vi "Device Params from Config INI File.vi"(8 "error in":errorcluster, 11 "Configuration in":refnum<class "Configuration.lvclass">) -> (0 "error out":errorcluster, 1 "Device Connections":T5={"PID Connections"={"Integrator DAQ Channels"={"V0"="cDAQ1Mod1/ai0", "S1"="cDAQ1Mod5/port0/line4", "S2"="cDAQ1Mod5/ctr0"}}, "Valve Controller VISA resource name"="COM3", "Detector Connection"=FALSE, "Power Supply Connection"=FALSE, "MFC Connection"=FALSE, "Valve Connection"=FALSE}, 2 "Device Settings":T8, 3 "Configuration out":refnum<class "Configuration.lvclass">)   [LabVIEW 2011]
uses:
  Modules/File/Configuration/Configuration.lvclass
  Controls/Device Settings.ctl
  Modules/Hardware/Power Supply/Source Units.ctl
  Modules/Hardware/Power Supply/Power Supply.lvclass
  Modules/Hardware/Power Supply/Source Mode.ctl
  Modules/Hardware/Mass Flow Controller/Valve Status.ctl
  Modules/Hardware/Mass Flow Controller/Mass Flow Controller.lvclass
  Modules/Hardware/Power Supply/Current Units.ctl
  Modules/Hardware/Power Supply/Voltage Units.ctl
  Modules/Hardware/Power Supply/Protection Limits.ctl
  Modules/Hardware/PID/Integrator DAQmx Channels.ctl
  Modules/Hardware/PID/PID.lvclass
  Modules/Hardware/PID/PID Connections.ctl
  Controls/Device Connections.ctl
  Modules/Hardware/Valve Controller/Valve Assembly.ctl
  Modules/Hardware/Valve Controller/Valve Controller.lvclass
  Controls/Valve Type.ctl
  Modules/File/Configuration/Key Data Type.ctl
  Modules/File/Configuration/PID Keys.ctl
  Modules/File/Configuration/PID Sections.ctl
  Modules/File/Configuration/PID Key Types.ctl
panel:
  in  "Key Types":T1=[enum."I32", enum."I32", enum."I32", enum."I32", enum."I32", enum."I32", enum."I32", enum."I32", enum."I32", enum."I32", enum."Double", enum."Double", enum."Double", enum."Double", enum."Double", enum."Double", enum."Double", enum."Double", enum."Double", enum."Boolean", enum."Boolean", enum."Boolean", enum."DAQmx Channel", enum."DAQmx Channel", enum."DAQmx Channel"]
  in  "Sections":T3=["Devices", "Devices", "Devices", "Devices", "Devices", "Devices", "Devices", "Devices", "Devices", "Devices", "Devices", "Devices", "Devices", "Devices", "Devices", "Devices", "Devices", "Devices", "Devices", "Devices", "Devices", "Devices", "Device Connections", "Device Connections", "Device Connections"]
  in  "Keys":T4=["Detector type", "MFC Type", "PS Type", "PS Source Units", "PS Source Mode", "MFC Valve Status", "PS Voltage Limit Units", "PS Current Limit Units", "PS Voltage Trip/Cmpl Units", "PS Current Trip/Cmpl Units", "PS Source Value", "MFC Flow Rate", "Detector Sampling Frequency", "PS Voltage Limit", "PS Current Limit", "PS Voltage Trip/Cmpl", "PS Current Trip/Cmpl", "PID Grid Voltage", "PID Integration Time", "Detector Connection", "MFC Connection", "PS Connection", "PID Integrator DAQmx Channel V0", "PID Integrator DAQmx Channel S1", "PID Integrator DAQmx Channel S2"]
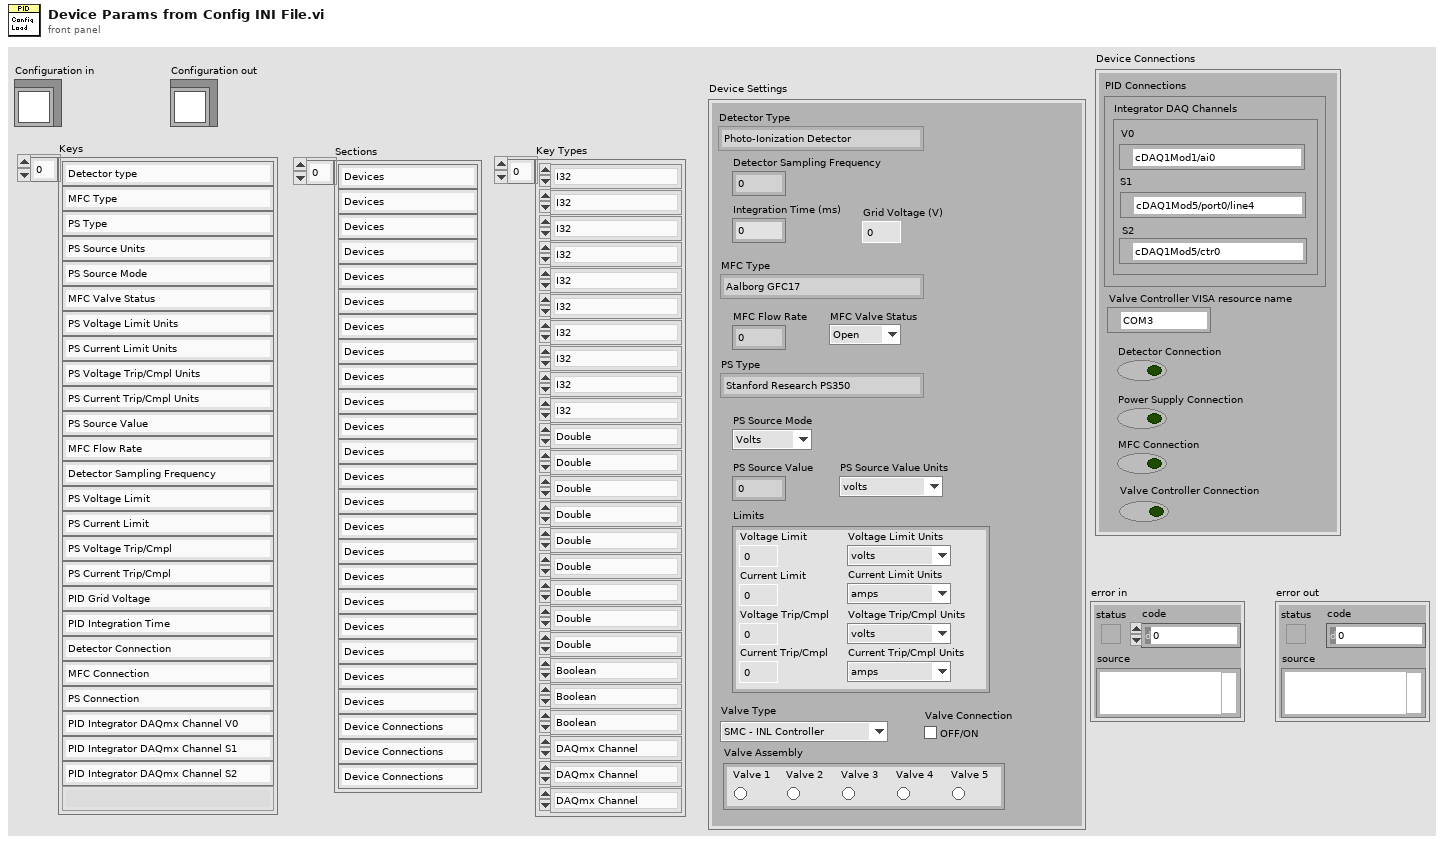
[diagram p1: front panel]
types:
  T1 = typedef "Configuration.lvclass/PID Key Types.ctl" = T2[]
  T2 = typedef "Configuration.lvclass/Key Data Type.ctl" = enum16{"Boolean", "U32", "I32", "Double", "String", "DAQmx Channel", "Path"}
  T3 = typedef "Configuration.lvclass/PID Sections.ctl" = string[]
  T4 = typedef "Configuration.lvclass/PID Keys.ctl" = string[]
  T5 = typedef "Device Connections.ctl" = cluster{"PID Connections":T6, "Valve Controller VISA resource name":refnum<visa-resource-name>, "Detector Connection":bool, "Power Supply Connection":bool, "MFC Connection":bool, "Valve Connection":bool}
  T6 = typedef "PID.lvclass/PID Connections.ctl" = cluster{"Integrator DAQ Channels":T7}
  T7 = typedef "PID.lvclass/Integrator DAQmx Channels.ctl" = cluster{"V0":tag, "S1":tag, "S2":tag}
  T8 = typedef "Device Settings.ctl" = cluster{"Detector Type":enum16{"Photo-Ionization Detector"}, "MFC Type":enum16{"Aalborg GFC17"}, "PS Type":enum16{"Stanford Research PS350", "Keithley 2400"}, "Detector Sampling Frequency":dbl, "MFC Flow Rate":dbl, "MFC Valve Status":T9, "PS Source Mode":T10, "PS Source Value":dbl, "PS Source Value Units":T11, "Limits":T12, "PID Integration Time":dbl, "PID Grid Voltage":dbl, "Valve Type":T15, "Valve Assembly":T16, "Valve Connection":bool}
  T9 = typedef "Mass Flow Controller.lvclass/Valve Status.ctl" = enum16{"Open", "Closed"}
  T10 = typedef "Power Supply.lvclass/Source Mode.ctl" = enum16{"Volts", "Current"}
  T11 = typedef "Power Supply.lvclass/Source Units.ctl" = enum16{"volts", "millivolts", "microvolts", "amps", "milliamps", "microamps", "nanoamps"}
  T12 = typedef "Power Supply.lvclass/Protection Limits.ctl" = cluster{"Voltage Limit":dbl, "Voltage Limit Units":T13, "Current Limit":dbl, "Current Limit Units":T14, "Voltage Trip/Cmpl":dbl, "Voltage Trip/Cmpl Units":T13, "Current Trip/Cmpl":dbl, "Current Trip/Cmpl Units":T14}
  T13 = typedef "Power Supply.lvclass/Voltage Units.ctl" = enum16{"volts", "millivolts", "microvolts"}
  T14 = typedef "Power Supply.lvclass/Current Units.ctl" = enum16{"amps", "milliamps", "microamps", "nanoamps"}
  T15 = typedef "Valve Type.ctl" = enum16{"SMC - INL Controller"}
  T16 = typedef "Valve Controller.lvclass/Valve Assembly.ctl" = cluster{"Valve 1":bool, "Valve 2":bool, "Valve 3":bool, "Valve 4":bool, "Valve 5":bool}
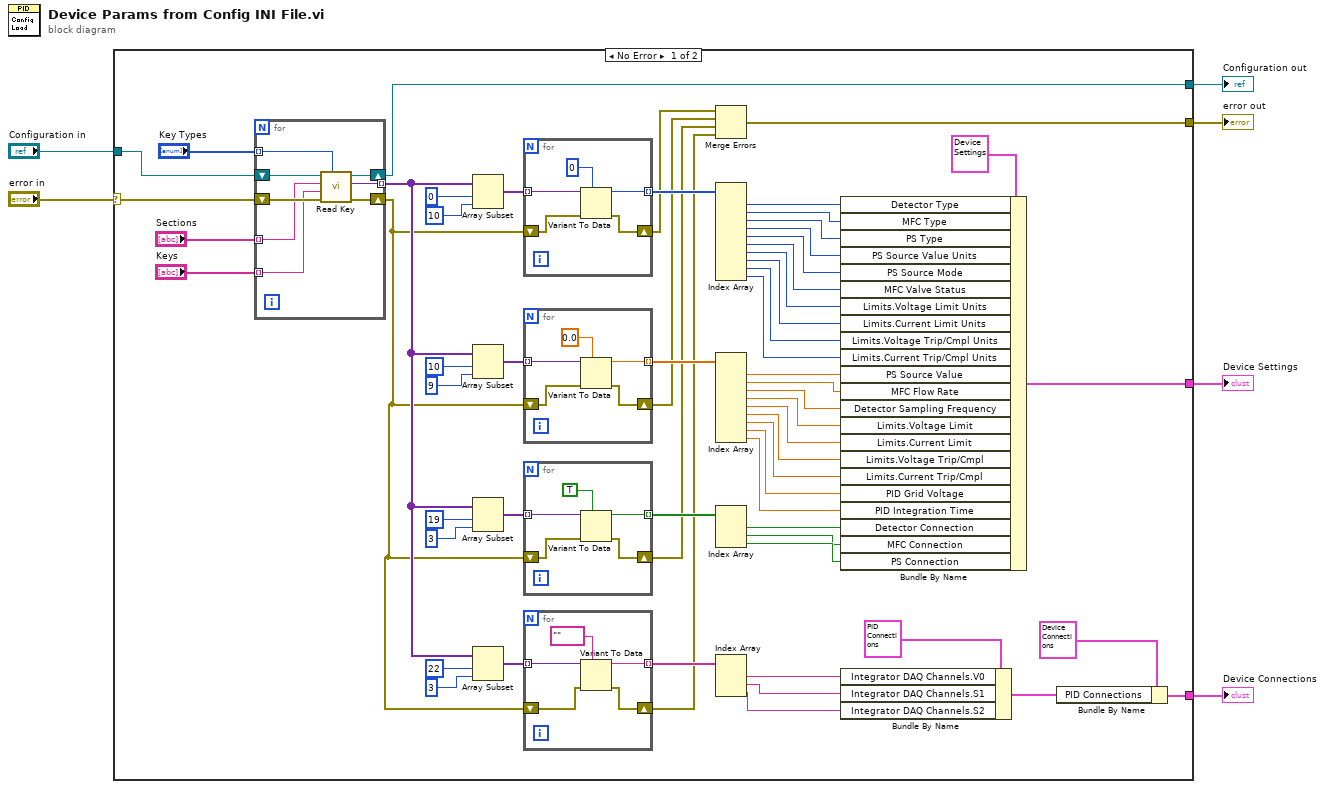
[diagram p0: block diagram]
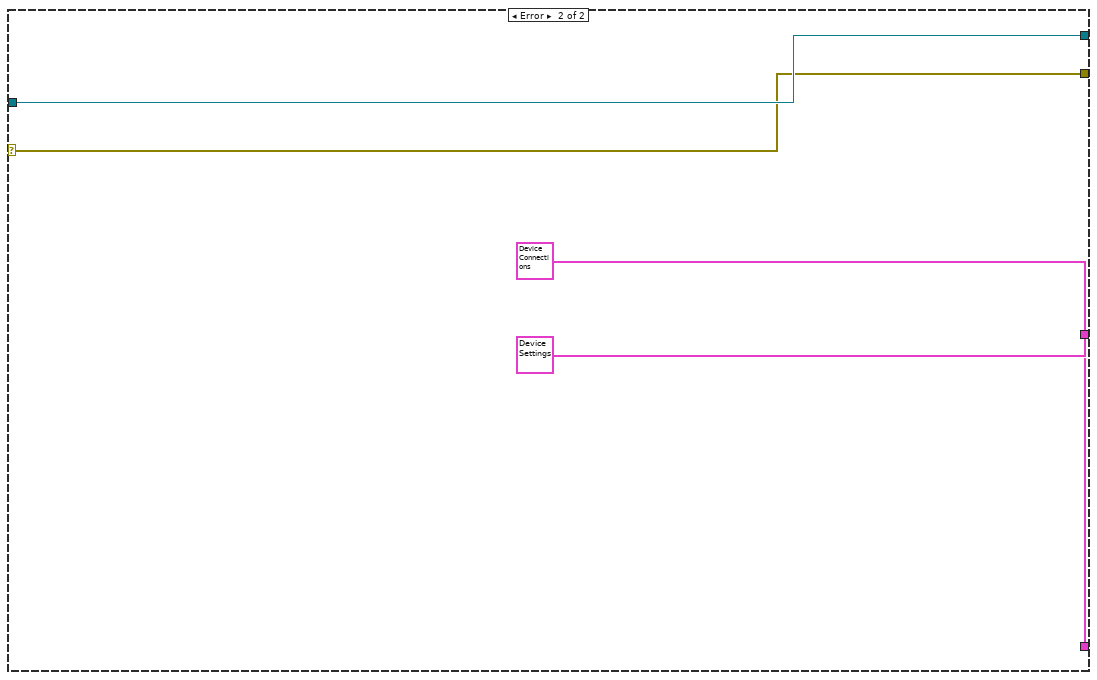
[diagram p2: hidden frame]
diagram:
  n1 = case shown="No Error" "error in" {
    selector: "error in" -> [w66 w97]
    tunnel: [w9 w98] -> w6
    tunnel: "Configuration in" -> [w65 w98]
    tunnel: [w10 w97] -> w4
    tunnel: [w8 T8 {"Detector Type"=enum."Photo-Ionization Detector", "MFC Type"=enum."Aalborg GFC17", "PS Type"=enum."Stanford Research PS350", "Detector Sampling Frequency"=0.0, "MFC Flow Rate"=0.0, "MFC Valve Status"=enum."Open", "PS Source Mode"=enum."Volts", "PS Source Value"=0.0, "PS Source Value Units"=enum."volts", "Limits"={"Voltage Limit"=0.0, "Voltage Limit Units"=enum."volts", "Current Limit"=0.0, "Current Limit Units"=enum."amps", "Voltage Trip/Cmpl"=0.0, "Voltage Trip/Cmpl Units"=enum."volts", "Current Trip/Cmpl"=0.0, "Current Trip/Cmpl Units"=enum."amps"}, "PID Integration Time"=0.0, "PID Grid Voltage"=0.0, "Valve Type"=enum."SMC - INL Controller", "Valve Assembly"={"Valve 1"=FALSE, "Valve 2"=FALSE, "Valve 3"=FALSE, "Valve 4"=FALSE, "Valve 5"=FALSE}, "Valve Connection"=FALSE} ("Device Settings")] -> w2
    tunnel: [w7 T5 {"PID Connections"={"Integrator DAQ Channels"={"V0"="cDAQ1Mod1/ai0", "S1"="cDAQ1Mod5/port0/line4", "S2"="cDAQ1Mod5/ctr0"}}, "Valve Controller VISA resource name"="", "Detector Connection"=FALSE, "Power Supply Connection"=FALSE, "MFC Connection"=FALSE, "Valve Connection"=FALSE} ("Device Connections")] -> w1
    frame No Error {
      n2 = for {
        shift-right: [w93] -> w9
        shift-left: w65 -> [w94]
        shift-right: [w87] -> w15
        shift-left: w66 -> [w92]
        tunnel: [w91] -> w23 mode=indexing
        tunnel: "Sections" -> [w90] mode=indexing
        tunnel: "Keys" -> [w89] mode=indexing
        tunnel: "Key Types" -> [w88] mode=indexing
        n3 = call-dynamic "Read Key.vi"("data type"=w88, "error in (no error)"=w92, "key"=w89, "section"=w90, "Configuration.lvclass in"=w94) -> ("error out"=w87:errorcluster, "Key"=w91:variant, "Configuration.lvclass out"=w93:refnum<class "Configuration.lvclass">)  [unwired: 3 in, 1 out]
      }
      n4 = Array Subset(array=w23, index=0, length=10) -> (w58:variant[])
      n5 = Array Subset(array=w23, index=10, length=9) -> (w44:variant[])
      n6 = Array Subset(array=w23, index=19, length=3) -> (w31:variant[])
      n7 = Array Subset(array=w23, index=22, length=3) -> (w24:variant[])
      n8 = for {
        tunnel: w58 -> [w86] mode=indexing
        tunnel: [w84] -> w57 mode=indexing
        shift-right: [w82] -> w14
        shift-left: w15 -> [w83]
        n9 = Variant To Data(error in=w83, type=0, Variant=w86) -> (data=w84:i32, error out=w82:errorcluster)
      }
      n10 = for {
        tunnel: w44 -> [w81] mode=indexing
        tunnel: [w79] -> w43 mode=indexing
        shift-right: [w77] -> w13
        shift-left: w15 -> [w78]
        n11 = Variant To Data(error in=w78, type=0.0, Variant=w81) -> (data=w79:dbl, error out=w77:errorcluster)
      }
      n12 = for {
        tunnel: w31 -> [w76] mode=indexing
        tunnel: [w75] -> w30 mode=indexing
        shift-right: [w72] -> w12
        shift-left: w15 -> [w73]
        n13 = Variant To Data(error in=w73, type=TRUE, Variant=w76) -> (data=w75:bool, error out=w72:errorcluster)
      }
      n14 = for {
        tunnel: w24 -> [w71] mode=indexing
        tunnel: [w70] -> w20 mode=indexing
        shift-right: [w67] -> w11
        shift-left: w15 -> [w68]
        n15 = Variant To Data(error in=w68, type=tag "" ("Integrator DAQ Channels.V0"), Variant=w71) -> (data=w70:tag, error out=w67:errorcluster)
      }
      n16 = Merge Errors(w14, w13, w12, w11) -> (w10:errorcluster)
      n17 = Index Array(array=w57) -> (element #1=w56:i32, element #2=w55:i32, element #3=w54:i32, element #4=w53:i32, element #5=w47:i32, element #6=w48:i32, element #7=w49:i32, element #8=w50:i32, element #9=w51:i32, element #10=w52:i32)  [unwired: 10 in]
      n18 = Index Array(array=w43) -> (element #1=w42:dbl, element #2=w41:dbl, element #3=w34:dbl, element #4=w35:dbl, element #5=w36:dbl, element #6=w37:dbl, element #7=w38:dbl, element #8=w39:dbl, element #9=w40:dbl)  [unwired: 9 in]
      n19 = Index Array(array=w30) -> (element #1=w29:bool, element #2=w27:bool, element #3=w28:bool)  [unwired: 3 in]
      n20 = Index Array(array=w20) -> (element #1=w19:tag, element #2=w17:tag, element #3=w18:tag)  [unwired: 3 in]
      n21 = Bundle By Name(cluster=T8 {"Detector Type"=enum."Photo-Ionization Detector", "MFC Type"=enum."Aalborg GFC17", "PS Type"=enum."Stanford Research PS350", "Detector Sampling Frequency"=0.0, "MFC Flow Rate"=0.0, "MFC Valve Status"=enum."Open", "PS Source Mode"=enum."Volts", "PS Source Value"=0.0, "PS Source Value Units"=enum."volts", "Limits"={"Voltage Limit"=0.0, "Voltage Limit Units"=enum."volts", "Current Limit"=0.0, "Current Limit Units"=enum."amps", "Voltage Trip/Cmpl"=0.0, "Voltage Trip/Cmpl Units"=enum."volts", "Current Trip/Cmpl"=0.0, "Current Trip/Cmpl Units"=enum."amps"}, "PID Integration Time"=0.0, "PID Grid Voltage"=0.0, "Valve Type"=enum."SMC - INL Controller", "Valve Assembly"={"Valve 1"=FALSE, "Valve 2"=FALSE, "Valve 3"=FALSE, "Valve 4"=FALSE, "Valve 5"=FALSE}, "Valve Connection"=FALSE} ("Device Settings"), "Detector Type"=w56, "MFC Type"=w55, "PS Type"=w54, "PS Source Value Units"=w53, "PS Source Mode"=w47, "MFC Valve Status"=w48, "Limits.Voltage Limit Units"=w49, "Limits.Current Limit Units"=w50, "Limits.Voltage Trip/Cmpl Units"=w51, "Limits.Current Trip/Cmpl Units"=w52, "PS Source Value"=w42, "MFC Flow Rate"=w41, "Detector Sampling Frequency"=w34, "Limits.Voltage Limit"=w35, "Limits.Current Limit"=w36, "Limits.Voltage Trip/Cmpl"=w37, "Limits.Current Trip/Cmpl"=w38, "PID Grid Voltage"=w39, "PID Integration Time"=w40, "Detector Connection"=w29, "MFC Connection"=w27, "PS Connection"=w28) -> (w8:T8)
      n22 = Bundle By Name(cluster=T6 {"Integrator DAQ Channels"={"V0"="cDAQ1Mod1/ai0", "S1"="cDAQ1Mod5/port0/line4", "S2"="cDAQ1Mod5/ctr0"}} ("PID Connections"), "Integrator DAQ Channels.V0"=w19, "Integrator DAQ Channels.S1"=w17, "Integrator DAQ Channels.S2"=w18) -> (w16:T6)
      n23 = Bundle By Name(cluster=T5 {"PID Connections"={"Integrator DAQ Channels"={"V0"="cDAQ1Mod1/ai0", "S1"="cDAQ1Mod5/port0/line4", "S2"="cDAQ1Mod5/ctr0"}}, "Valve Controller VISA resource name"="", "Detector Connection"=FALSE, "Power Supply Connection"=FALSE, "MFC Connection"=FALSE, "Valve Connection"=FALSE} ("Device Connections"), "PID Connections"=w16) -> (w7:T5)
    }
    frame Error {
    }
  }
  "Configuration out" <- w6
  "error out" <- w4
  "Device Settings" <- w2
  "Device Connections" <- w1
